vi "Main.vi"() -> ()   [LabVIEW 2020]
doc: "This template is for the Queued Message Handler design pattern.\n\nThe Event Handling Loop generates messages based on user interface actions.\n\nThe Message Handling Loop processes messages generated by the Event Handling Loop, or by other messages. The messages are string values, so new messages can be added easily to the Message Cases case structure in the Message Handling Loop. Each message cluster can also provide an optional value for Message Data, which is a variant that can be converted to whatever message-specific data is required."
uses:
  <vilib>/userdefined/High Color/IMAQdx.ctl
  controls/UI Data.ctl
  support/Message Queue/Enqueue Message (Single).vi
  <vilib>/addons/database/Connection.llb/DB Tools Open Connec (Path).vi
  <vilib>/Utility/error.llb/Error Cluster From Error Code.vi
  <vilib>/ErrorRing/Error Ring.xnode
  support/Message Queue/Message Queue.lvlib
  support/User Event - Stop/User Event - Stop.lvlib
  <vilib>/vision/driver/NI_Vision_Acquisition_Software.lvlib
  <vilib>/addons/database/NI_Database_API.lvlib
panel:
  in  "Save Results in DB":bool
  in  "DB connection file":path
  out "Face Mask":bool
  in  "Camera channel":T1
  out "Image":T2(plugin-control)
  out "Display":string
  in  "Stop Recording":bool
  in  "Start Recording":bool
  in  "Exit":bool
  # "Choose Camera Input"
  # "Choose Database Connection File"
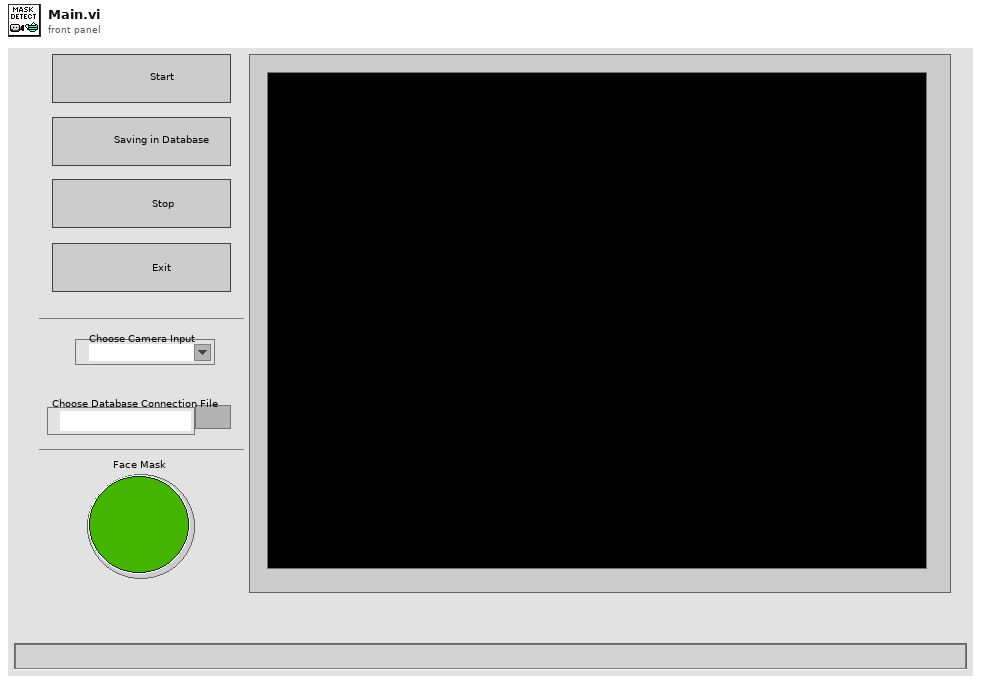
[diagram p1: front panel]
types:
  T1 = typedef "IMAQdx.ctl" = refnum<k21>
  T2 = typedef "IMAQ Image.ctl" = refnum<image>
  T3 = typedef "UI Data.ctl" = cluster{"Start Recording Ref":refnum<vi>, "Stop Recording Ref":refnum<vi>, "Display Ref":refnum<vi>, "Exit  Ref":refnum<vi>, "status ":string, "CAM channel":refnum<vi>}
  T4 = typedef "Message Queue.lvlib/All Message Queues.ctl" = cluster{"UI":refnum<queue>, "Recording ":refnum<queue>}
  T5 = typedef "Image Type" = u32
  T6 = typedef "NI_Database_API.lvlib/Conn ObjectReference.ctl" = refnum<k1>
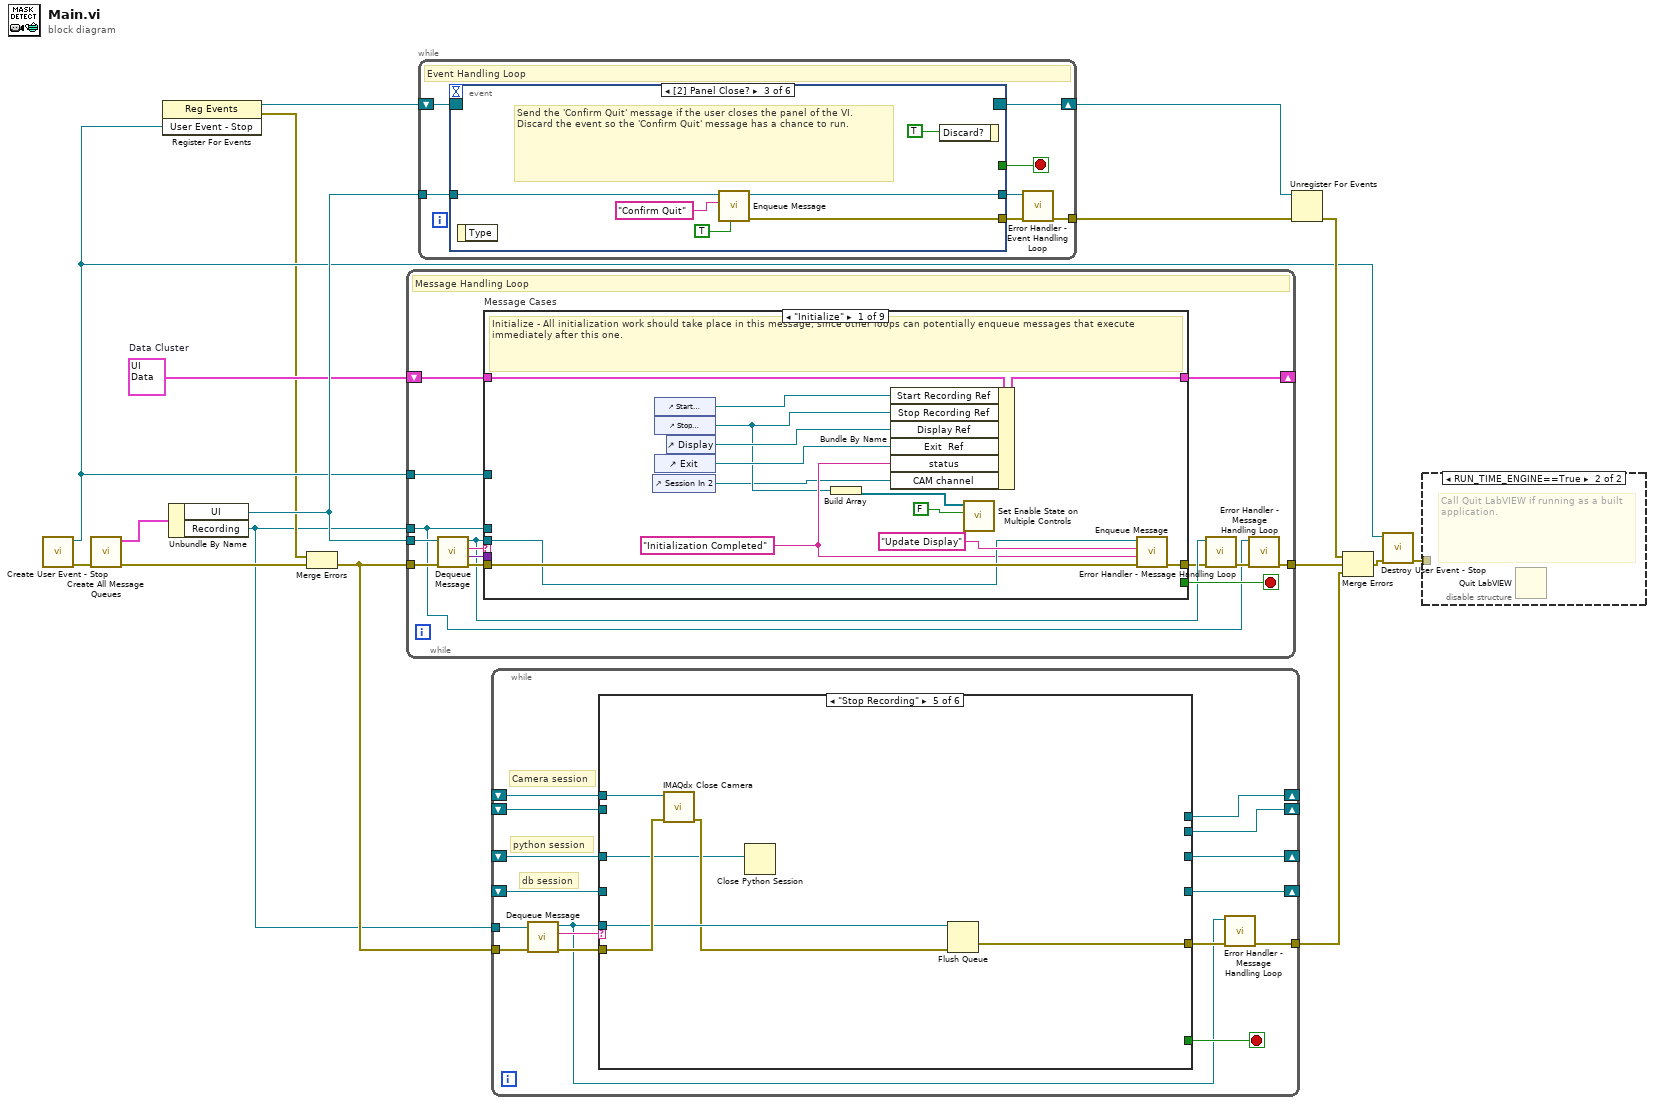
[diagram p0: block diagram]
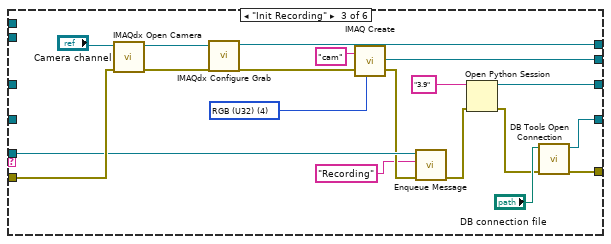
[diagram p4: hidden frame]
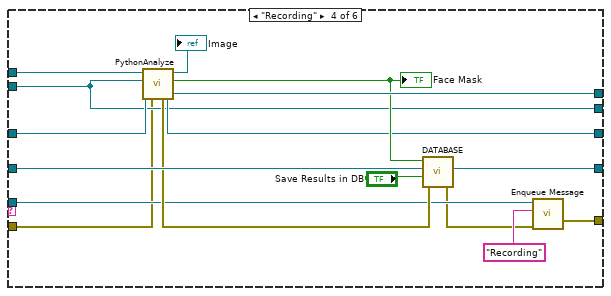
[diagram p5: hidden frame]
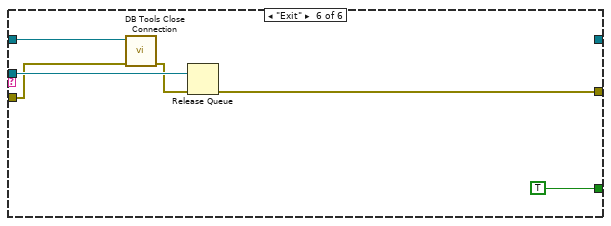
[diagram p6: hidden frame]
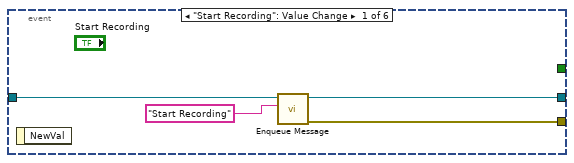
[diagram p8: hidden frame]
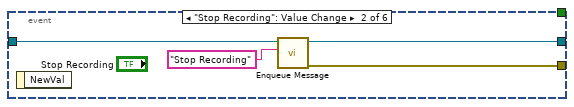
[diagram p9: hidden frame]
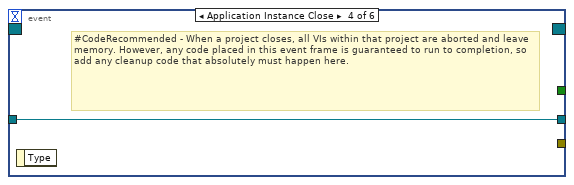
[diagram p10: hidden frame]
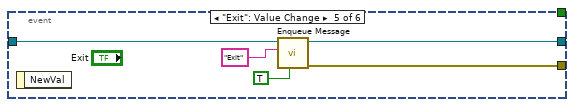
[diagram p11: hidden frame]
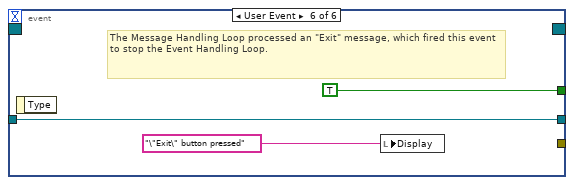
[diagram p12: hidden frame]
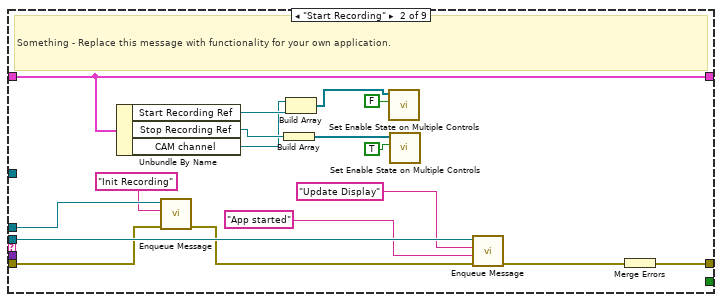
[diagram p13: hidden frame]
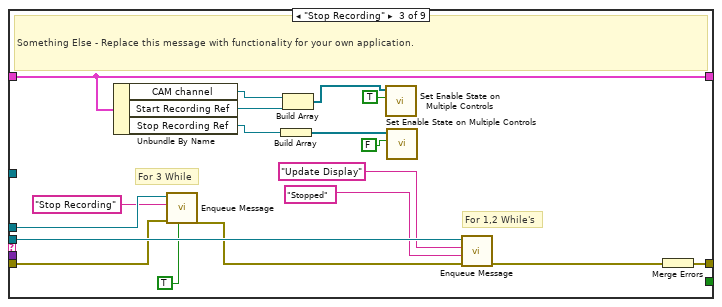
[diagram p14: hidden frame]
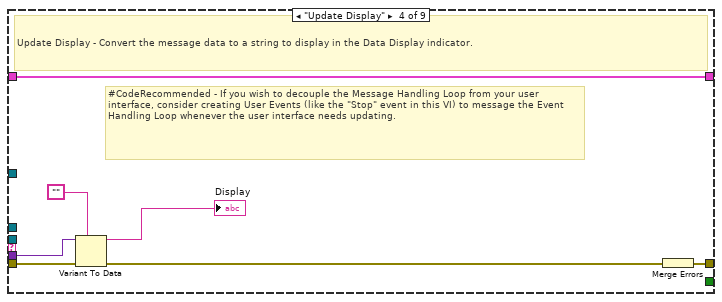
[diagram p15: hidden frame]
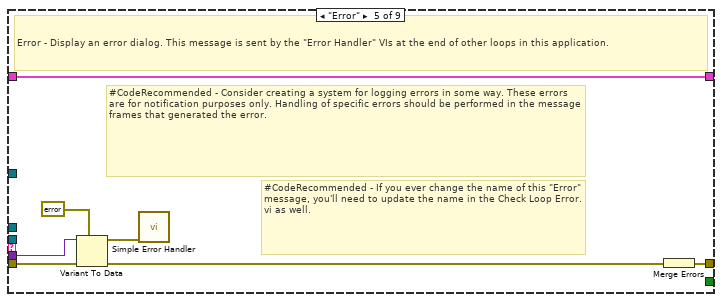
[diagram p16: hidden frame]
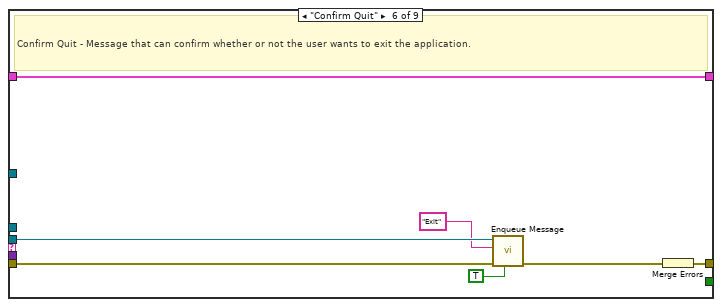
[diagram p17: hidden frame]
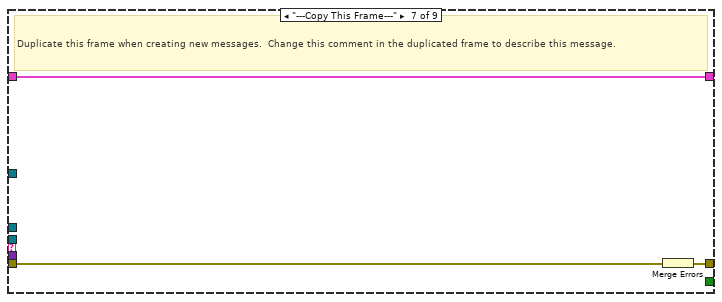
[diagram p18: hidden frame]
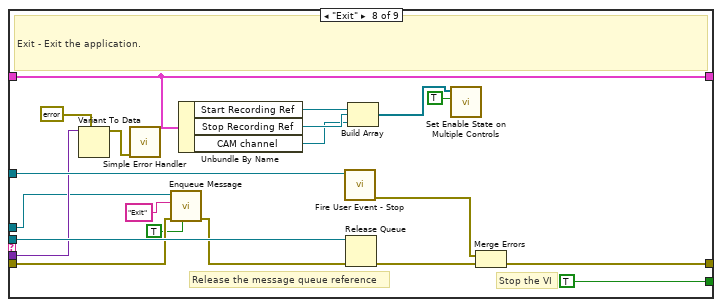
[diagram p19: hidden frame]
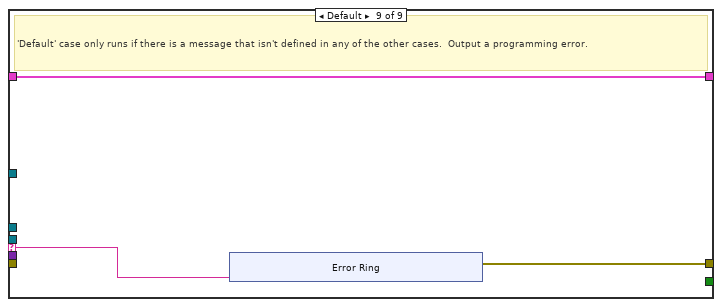
[diagram p20: hidden frame]
diagram:
  w9 = T3 {"Start Recording Ref"=refnum, "Stop Recording Ref"=refnum, "Display Ref"=refnum, "Exit  Ref"=refnum, "status "="", "CAM channel"=refnum}  # Data Cluster
  n1 = call "Create User Event - Stop.vi"() -> ("error out"=w13:errorcluster, "User Event - Stop"=w5:refnum<user-event>)  [unwired: 10 in]
  n2 = call "Create All Message Queues.vi"("error in (no error)"=w13) -> ("error out"=w17:errorcluster, "Message Queues out"=w16:T4)  [unwired: 9 in]
  n3 = register-events(w5) -> (reference out=w6:refnum<event-registration>, error out=w4:errorcluster)  [unwired: 2 in]
  n4 = Unbundle By Name(w16) -> ("UI"=w14:refnum<queue>, "Recording"=w2:refnum<queue>)
  n5 = Merge Errors(w4, w17) -> (w3:errorcluster)
  n6 = while {
    tunnel: w14 -> [w23]
    shift-right: [w30] -> _
    shift-left: w9 -> [w31]
    tunnel: w5 -> [w28]
    tunnel: w3 -> [w27]
    tunnel: [w19] -> w15
    tunnel: w2 -> [w18]
    stop <- w29 stop-if-true
    # "Message Handling Loop"
    n7 = call "Dequeue Message.vi"("error in (no error)"=w27, "Message Queue"=w23) -> ("error out"=w26:errorcluster, "Message Data"=w24:variant, "Message"=w25:string, "dup Message Queue"=w22:refnum<queue>)  [unwired: 6 in]
    n8 = case "Message Cases" shown="\"Initialize\"" w25 {
      selector: w25 -> [_ _ _ _ _ _ _ _ w125]
      tunnel: w22 -> [w38 w60 w78 _ _ w97 _ w124 _]
      tunnel: w26 -> [w44 w48 w65 w85 w94 w101 w104 w108 _]
      tunnel: [w45 w62 w80 w86 w88 w99 w102 w121 w126] -> w21
      tunnel: w31 -> [w43 w57 w70 w87 w93 w100 w103 w111 w127]
      tunnel: [w42 w57 w70 w87 w93 w100 w103 w111 w127] -> w30
      tunnel: [_ _ _ _ _ _ _ TRUE _] -> w29
      tunnel: w24 -> [_ _ _ w84 w92 _ _ w116 _]
      tunnel: w28 -> [_ _ _ _ _ _ _ w120 _]
      tunnel: w18 -> [_ w50 w68 _ _ _ _ w110 _]
      frame "Initialize" {
        w37 = "Initialization Completed" ("Initial Message")
        # "Initialize - All initialization work should take place in this message, since other loops can potentially enqueue messages that execute immediately after this one."
        n9 = control-ref of="Session In 2"() -> (w32:refnum<vi>)
        n10 = control-ref of="Start Recording"() -> (w33:refnum<vi>)
        n11 = control-ref of="Stop Recording"() -> (w34:refnum<vi>)
        n12 = control-ref of="Exit"() -> (w40:refnum<vi>)
        n13 = control-ref of="Display"() -> (w41:refnum<vi>)
        n14 = Build Array(w34) -> (w35:refnum<vi>[])
        n15 = Bundle By Name(cluster=w43, "Start Recording Ref"=w33, "Stop Recording Ref"=w34, "Display Ref"=w41, "Exit  Ref"=w40, "status"=w37, "CAM channel"=w32) -> (w42:T3)
        n16 = call "Set Enable State on Multiple Controls.vi"("Enable?"=FALSE, "Controls"=w35) -> ()  [unwired: 10 in]
        n17 = call-poly "Enqueue Message.vi"("error in (no error)"=w44, "Message Data"=w37, "Message"="Update Display", "Message Queue"=w38) -> ("error out"=w45:errorcluster)  [unwired: 6 in, 1 out]
      }
      frame "Start Recording" {
        # "Something - Replace this message with functionality for your own application."
        n18 = Unbundle By Name(w57) -> ("Start Recording Ref"=w54:refnum<vi>, "Stop Recording Ref"=w52:refnum<vi>, "CAM channel"=w46:refnum<vi>)
        n19 = call-poly "Enqueue Message.vi"("error in (no error)"=w48, "Message"="Init Recording", "Message Queue"=w50) -> ("error out"=w47:errorcluster)  [unwired: 7 in, 1 out]
        n20 = Build Array(w52) -> (w51:refnum<vi>[])
        n21 = Build Array(w46, w54) -> (w53:refnum<vi>[])
        n22 = call "Set Enable State on Multiple Controls.vi"("Enable?"=FALSE, "Controls"=w53) -> ()  [unwired: 10 in]
        n23 = call "Set Enable State on Multiple Controls.vi"("Enable?"=TRUE, "Controls"=w51) -> ()  [unwired: 10 in]
        n24 = call-poly "Enqueue Message.vi"("error in (no error)"=w47, "Message Data"="App started" ("\"Do Something\" button pressed"), "Message"="Update Display", "Message Queue"=w60) -> ("error out"=w61:errorcluster)  [unwired: 6 in, 1 out]
        n25 = Merge Errors(w61) -> (w62:errorcluster)
      }
      frame "Stop Recording" {
        # "For 1,2 While's"
        # "For 3 While"
        # "Something Else - Replace this message with functionality for your own application."
        n26 = Unbundle By Name(w70) -> ("CAM channel"=w63:refnum<vi>, "Start Recording Ref"=w73:refnum<vi>, "Stop Recording Ref"=w72:refnum<vi>)
        n27 = call-poly "Enqueue Message.vi"("Priority Message? (F)"=TRUE, "error in (no error)"=w65, "Message"="Stop Recording", "Message Queue"=w68) -> ("error out"=w64:errorcluster)  [unwired: 6 in, 1 out]
        n28 = Build Array(w72) -> (w71:refnum<vi>[])
        n29 = Build Array(w63, w73) -> (w69:refnum<vi>[])
        n30 = call "Set Enable State on Multiple Controls.vi"("Enable?"=TRUE, "Controls"=w69) -> ()  [unwired: 10 in]
        n31 = call "Set Enable State on Multiple Controls.vi"("Enable?"=FALSE, "Controls"=w71) -> ()  [unwired: 10 in]
        n32 = call-poly "Enqueue Message.vi"("error in (no error)"=w64, "Message Data"="Stopped" ("\"Do Something Else\" button pressed"), "Message"="Update Display", "Message Queue"=w78) -> ("error out"=w79:errorcluster)  [unwired: 6 in, 1 out]
        n33 = Merge Errors(w79) -> (w80:errorcluster)
      }
      frame "Update Display" {
        # "#CodeRecommended - If you wish to decouple the Message Handling Loop from your user interface, consider creating User Events (like the \"Stop\" event in this VI) to message the Event Handling Loop whenever the user interface needs updating."
        # "Update Display - Convert the message data to a string to display in the Data Display indicator."
        n34 = Variant To Data(error in=w85, type="" ("Empty String Constant"), Variant=w84) -> (data=→"Display":string, error out=w82:errorcluster)
        n35 = Merge Errors(w82) -> (w86:errorcluster)
      }
      frame "Error" {
        # "#CodeRecommended - If you ever change the name of this \"Error\" message, you'll need to update the name in the Check Loop Error.vi as well."
        # "#CodeRecommended - Consider creating a system for logging errors in some way. These errors are for notification purposes only. Handling of specific errors should be performed in the message frames that generated the error."
        # "Error - Display an error dialog. This message is sent by the \"Error Handler\" VIs at the end of other loops in this application."
        n36 = Variant To Data(error in=w94, type=errorcluster {"status"=FALSE, "code"=0, "source"=""} ("error constant"), Variant=w92) -> (data=w90:errorcluster, error out=w89:errorcluster)
        n37 = call <vilib>:"Simple Error Handler.vi"("error in (no error)"=w90) -> ()  [unwired: 4 in, 5 out]
        n38 = Merge Errors(w89) -> (w88:errorcluster)
      }
      frame "Confirm Quit" {
        # "Confirm Quit - Message that can confirm whether or not the user wants to exit the application."
        n39 = call-poly "Enqueue Message.vi"("Priority Message? (F)"=TRUE, "error in (no error)"=w101, "Message"="Exit", "Message Queue"=w97) -> ("error out"=w98:errorcluster)  [unwired: 6 in, 1 out]
        n40 = Merge Errors(w98) -> (w99:errorcluster)
      }
      frame "---Copy This Frame---" {
        # "Duplicate this frame when creating new messages.  Change this comment in the duplicated frame to describe this message."
        n41 = Merge Errors(w104) -> (w102:errorcluster)
      }
      frame "Exit" {
        # "Stop the VI"
        # "Release the message queue reference"
        # "Exit - Exit the application."
        n42 = Variant To Data(type=errorcluster {"status"=FALSE, "code"=0, "source"=""} ("error constant"), Variant=w116) -> (data=w117:errorcluster)  [unwired: 1 in, 1 out]
        n43 = call <vilib>:"Simple Error Handler.vi"("error in (no error)"=w117) -> ()  [unwired: 4 in, 5 out]
        n44 = call-poly "Enqueue Message.vi"("Priority Message? (F)"=TRUE, "error in (no error)"=w108, "Message"="Exit", "Message Queue"=w110) -> ("error out"=w107:errorcluster)  [unwired: 6 in, 1 out]
        n45 = Unbundle By Name(w111) -> ("Start Recording Ref"=w114:refnum<vi>, "Stop Recording Ref"=w113:refnum<vi>, "CAM channel"=w105:refnum<vi>)
        n46 = call "Fire User Event - Stop.vi"("User Event - Stop"=w120) -> ("error out"=w119:errorcluster)  [unwired: 10 in]
        n47 = Release Queue(queue=w124, error in (no error)=w107) -> (error out=w122:errorcluster)  [unwired: 1 in, 2 out]
        n48 = Build Array(w114, w113, w105) -> (w112:refnum<vi>[])
        n49 = call "Set Enable State on Multiple Controls.vi"("Enable?"=TRUE, "Controls"=w112) -> ()  [unwired: 10 in]
        n50 = Merge Errors(w119, w122) -> (w121:errorcluster)
      }
      frame Default {
        # "'Default' case only runs if there is a message that isn't defined in any of the other cases.  Output a programming error."
        n51 = xnode ("Error Ring")("parameter 0"=w125) -> ("error out"=w126:errorcluster)
      }
    }
    n52 = call "Error Handler - Message Handling Loop.vi"("error in (no error)"=w21, "Message Queue"=w22) -> ("dup error in"=w20:errorcluster)  [unwired: 8 in, 1 out]
    n53 = call "Error Handler - Message Handling Loop.vi"("error in (no error)"=w20, "Message Queue"=w18) -> ("dup error in"=w19:errorcluster)  [unwired: 8 in, 1 out]
  }
  n54 = while {
    tunnel: w14 -> [w141]
    shift-right: [w139] -> w10
    shift-left: w6 -> [w140]
    tunnel: [w135] -> w7
    stop <- w137 stop-if-true
    # "Event Handling Loop"
    n55 = event shown="[2] Panel Close?" {
      selector: w140 -> [_ _ _ _ _ _]
      dyn-events: [_ _ _ _ _ _] -> w139
      timeout: _ -> [_ _ _ _ _ _]
      tunnel: [_ _ _ _ _ TRUE ("Discard?")] -> w137
      tunnel: w141 -> [w145 w149 w154 w156 w161 w164]
      tunnel: [w142 w146 w153 _ w160 _] -> w138
      tunnel: [w144 w148 w152 w156 w159 w164] -> w136
      event "Start Recording": Value Change {
        n56 = event-data() -> ()  [unwired: 1 in, 1 out]
        n57 = call-poly "Enqueue Message.vi"("Message"="Start Recording", "Message Queue"=w145) -> ("error out"=w142:errorcluster, "dup Message Queue"=w144:refnum<queue>)  [unwired: 8 in]
      }
      event "Stop Recording": Value Change {
        n58 = event-data() -> ()  [unwired: 1 in, 1 out]
        n59 = call-poly "Enqueue Message.vi"("Message"="Stop Recording", "Message Queue"=w149) -> ("error out"=w146:errorcluster, "dup Message Queue"=w148:refnum<queue>)  [unwired: 8 in]
      }
      event Panel Close? {
        # "Send the 'Confirm Quit' message if the user closes the panel of the VI. Discard the event so the 'Confirm Quit' message has a chance to run."
        n60 = event-data() -> ()  [unwired: 1 in, 1 out]
        n61 = call-poly "Enqueue Message.vi"("Priority Message? (F)"=TRUE, "Message"="Confirm Quit", "Message Queue"=w154) -> ("error out"=w153:errorcluster, "dup Message Queue"=w152:refnum<queue>)  [unwired: 7 in]
        n62 = event-data ("Event Filter Node")("Discard?"=TRUE) -> ()  [unwired: 1 in, 1 out]
      }
      event Application Instance Close {
        # "#CodeRecommended - When a project closes, all VIs within that project are aborted and leave memory. However, any code placed in this event frame is guaranteed to run to completion, so add any cleanup code that absolutely must happen here."
        n63 = event-data() -> ()  [unwired: 1 in, 1 out]
      }
      event "Exit": Value Change {
        n64 = event-data() -> ()  [unwired: 1 in, 1 out]
        n65 = call-poly "Enqueue Message.vi"("Priority Message? (F)"=TRUE, "Message"="Exit", "Message Queue"=w161) -> ("error out"=w160:errorcluster, "dup Message Queue"=w159:refnum<queue>)  [unwired: 7 in]
      }
      event User Event {
        # "The Message Handling Loop processed an \"Exit\" message, which fired this event to stop the Event Handling Loop."
        n66 = event-data() -> ()  [unwired: 1 in, 1 out]
        n67 = local write "Display"("\"Exit\" button pressed" ("VI Stopped")) -> ()
      }
    }
    n68 = call "Error Handler - Event Handling Loop.vi"("error in (no error)"=w138, "Message Queue"=w136) -> ("dup error in"=w135:errorcluster)  [unwired: 8 in, 1 out]
  }
  n69 = while {
    tunnel: w2 -> [w180]
    tunnel: w3 -> [w178]
    tunnel: [w175] -> w1
    shift-right: [w172] -> _
    shift-left: _ -> [w170]
    shift-right: [w171] -> _
    shift-left: _ -> [w169]
    shift-right: [w168] -> _
    shift-left: _ -> [w167]
    shift-right: [w166] -> _
    shift-left: _ -> [w165]
    stop <- w174 stop-if-true
    # "db session"
    # "Camera session"
    # "python session"
    n70 = call "Dequeue Message.vi"("error in (no error)"=w178, "Message Queue"=w180) -> ("error out"=w177:errorcluster, "Message"=w179:string, "dup Message Queue"=w173:refnum<queue>)  [unwired: 6 in, 1 out]
    n71 = case shown="\"Stop Recording\"" w179 {
      tunnel: w173 -> [_ _ w196 w206 w222 w229]
      tunnel: w177 -> [w181 w182 w200 w204 w223 w225]
      tunnel: [w181 w182 w185 w202 w220 w228] -> w176
      tunnel: [_ _ _ _ _ TRUE] -> w174
      tunnel: [_ _ w198 w207 _ _] -> w171
      tunnel: [_ _ w197 w215 _ _] -> w172
      tunnel: w170 -> [_ _ _ w217 w219 _]
      tunnel: w169 -> [_ _ _ w207 _ _]
      tunnel: [_ _ w189 w208 _ _] -> w168
      tunnel: w167 -> [_ _ _ w216 w218 _]
      tunnel: [_ _ w186 w213 _ _] -> w166
      tunnel: w165 -> [_ _ _ w214 _ w226]
      frame "False", Default {
      }
      frame "Initialize" {
      }
      frame "Init Recording" {
        w193 = T5 4 items=["Grayscale (U8)", "Grayscale (I16)", "Grayscale (SGL)", "Complex (CSG)", "RGB (U32)", "HSL (U32)", "RGB (U64)", "Grayscale (U16)"] ("Image Type")
        n72 = call <vilib>:"IMAQdx Open Camera.vi"("error in"=w200, "Session In"="Camera channel") -> ("error out"=w192:errorcluster, "Session Out"=w188:T1)  [unwired: 8 in]
        n73 = call <vilib>:"IMAQdx Configure Grab.vi"("error in"=w192, "Session In"=w188) -> ("error out"=w199:errorcluster, "Session Out"=w197:T1)  [unwired: 8 in]
        n74 = call "IMAQ Create"("Image Name"="cam", "Image Type"=w193, "error in (no error)"=w199) -> ("New Image"=w198:T2, "error out"=w195:errorcluster)  [unwired: 2 in]
        n75 = call-poly "Enqueue Message.vi"("error in (no error)"=w195, "Message"="Recording", "Message Queue"=w196) -> ("error out"=w184:errorcluster)  [unwired: 7 in, 1 out]
        n76 = Open Python Session(python version="3.9" ("Python version"), 3:w184) -> (session out=w189:refnum<k35>, error out=w183:errorcluster)  [unwired: 1 in]
        n77 = call-poly <vilib>:"DB Tools Open Connection.vi"("error in (no error)"=w183, "connection information"="DB connection file") -> ("error out"=w185:errorcluster, "connection reference"=w186:T6)  [unwired: 6 in]
      }
      frame "Recording" {
        n78 = call "PythonAnalyze.vi"("error in (no error)"=w204, "Python Session In"=w216, "Frame Space"=w207, "Cam Session"=w217) -> ("Python session out 2"=w208:refnum<k35>, "Cam Session Out 2"=w215:T1, "Mask"=w211:bool, "Image Out"=→"Image":T2, "error out"=w209:errorcluster)  [unwired: 3 in]
        "Face Mask" <- w211
        n79 = call "DATABASE.vi"("error in (no error)"=w209, "saving"="Save Results in DB", "connection reference"=w214, "mask led"=w211) -> ("error out"=w203:errorcluster, "connection reference out"=w213:T6)  [unwired: 2 in]
        n80 = call-poly "Enqueue Message.vi"("error in (no error)"=w203, "Message"="Recording", "Message Queue"=w206) -> ("error out"=w202:errorcluster)  [unwired: 7 in, 1 out]
      }
      frame "Stop Recording" {
        n81 = call <vilib>:"IMAQdx Close Camera.vi"("error in"=w223, "Session In"=w219) -> ("error out"=w221:errorcluster)  [unwired: 9 in]
        n82 = Close Python Session(session in=w218) -> ()  [unwired: 1 in, 1 out]
        n83 = Flush Queue(queue=w222, error in (no error)=w221) -> (error out=w220:errorcluster)  [unwired: 2 out]
      }
      frame "Exit" {
        n84 = call <vilib>:"DB Tools Close Connection.vi"("error in (no error)"=w225, "connection reference"=w226) -> ("error out"=w224:errorcluster)  [unwired: 5 in]
        n85 = Release Queue(queue=w229, error in (no error)=w224) -> (error out=w228:errorcluster)  [unwired: 1 in, 2 out]
      }
    }
    n86 = call "Error Handler - Message Handling Loop.vi"("error in (no error)"=w176, "Message Queue"=w173) -> ("dup error in"=w175:errorcluster)  [unwired: 8 in, 1 out]
  }
  n87 = Unregister For Events(event registration refnum=w10, error in=w7) -> (error out=w11:errorcluster)
  n88 = Merge Errors(w11, w15, w1) -> (w12:errorcluster)
  n89 = call "Destroy User Event - Stop.vi"("error in (no error)"=w12, "User Event - Stop"=w5) -> ("error out"=w8:errorcluster)  [unwired: 9 in]
  n90 = disable-structure "Conditional Disable Structure" shown="RUN_TIME_ENGINE==True" {
    disable-tunnel: w8 -> [_ _]
    frame condition #0 (active) {
    }
    frame condition #1 {
      # "Call Quit LabVIEW if running as a built application."
      n91 = Quit LabVIEW() -> ()  [unwired: 1 in]
    }
  }
